vi "RSZVB Trace Assign Diagram Area.vi"(7 "Trace Name (Trc1)":string="Trc1", 8 "error in (no error)":errorcluster {"code" format="%.0x"}, 9 "Window (Trace) (1)":i32=1, 10 "Window (1)":i32=1, 11 "VISA session":refnum<visa-resource-name>) -> (0 "error out":errorcluster {"code" format="%.0x"}, 3 "dup VISA session":refnum<visa-resource-name>)   [LabVIEW 2011]
doc: "This VI assigns the active trace to another diagram area. Selecting one of the existing area numbers assigns the active trace to the existing diagram area: The active trace is removed from the previous area and displayed in the new diagram area.\n\nNote(s):\n\n(1) A trace can be assigned to a diagram only once. If a attempt is made to assign the same trace a second time an error message –114,\"Header suffix out of range\" is generated.\n\nRemote-control command(s):\nDISPlay:WINDow<Wnd>:TRACe<WndTr>:FEED <string>"
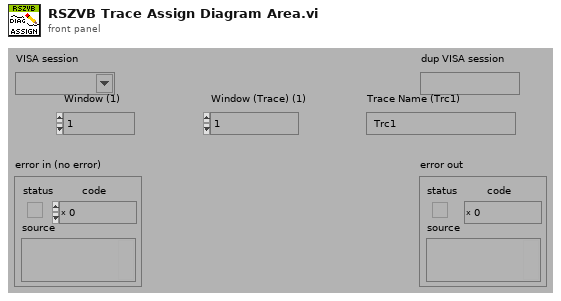
[diagram p1: front panel]
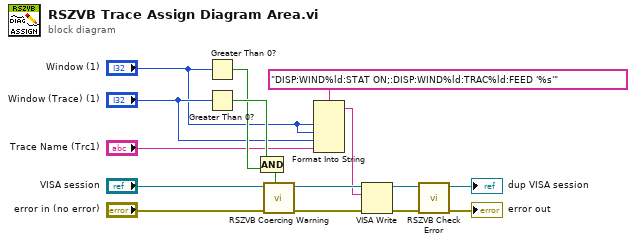
[diagram p0: block diagram]
diagram:
  n1 = Greater Than 0?(x="Window (1)") -> (x > 0?=w7:bool)
  n2 = Greater Than 0?(x="Window (Trace) (1)") -> (x > 0?=w8:bool)
  n3 = Compound Arithmetic op=AND(w8, w7) -> (w6:bool)
  n4 = call "RSZVB Coercing Warning.vi"("In Range?"=w6, "error in (no error)"="error in (no error)", "VISA session"="VISA session") -> ("error out"=w14:errorcluster, "dup VISA session"=w15:refnum<visa-resource-name>)  [unwired: 7 in]
  n5 = Format Into String(format string="DISP:WIND%ld:STAT ON;:DISP:WIND%ld:TRAC%ld:FEED '%s'", "Window (1)", "Window (1)", "Window (Trace) (1)", "Trace Name (Trc1)") -> (resulting string=w11:string)  [unwired: 2 in, 1 out]
  n6 = VISA Write(VISA resource name=w15, write buffer=w11, error in (no error)=w14) -> (VISA resource name out=w12:refnum<visa-resource-name>, error out=w13:errorcluster)  [unwired: 1 out]
  n7 = call "RSZVB Check Error.vi"("error in (no error)"=w13, "VISA session"=w12) -> ("error out"=→"error out":errorcluster, "dup VISA session"=→"dup VISA session":refnum<visa-resource-name>)  [unwired: 8 in]
